vi "triatge dades.vi"(8 "shift register left":string, 10 "dada a buscar":string=":", 11 "String in":string) -> (0 "shift register right":string, 1 "String Out":string, 2 "Data Out (string)":string, 3 "Data Out":dbl)   [LabVIEW 2018]
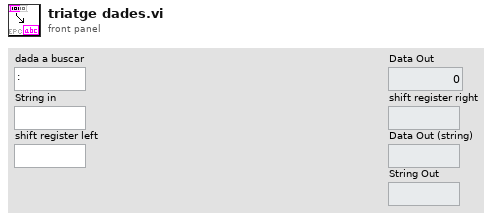
[diagram p1: front panel]
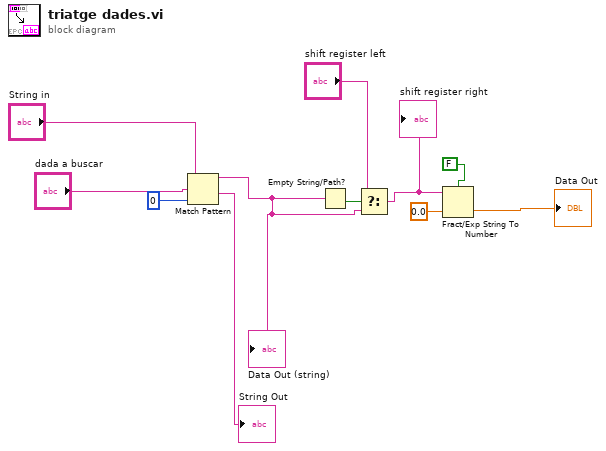
[diagram p0: block diagram]
diagram:
  n1 = Match Pattern(string="String in", regular expression="dada a buscar", offset (0)=0 ("t")) -> (before substring=w6:string, after substring=→"String Out":string)  [unwired: 2 out]
  "Data Out (string)" <- w6
  n2 = Empty String/Path?(string/path=w6) -> (empty?=w7:bool)
  n3 = Select(t="shift register left", s=w7, f=w6) -> (s? t:f=w8:string)
  "shift register right" <- w8
  n4 = Fract/Exp String To Number(use system decimal point (T)=FALSE, string=w8, default (0 dbl)=0.0) -> (number=→"Data Out":dbl)  [unwired: 1 in, 1 out]
